vi "Connect.vi"(8 "error in (no error)":errorcluster, 11 "Stepper3D in":refnum<class "Stepper3D.lvclass">) -> (0 "error out":errorcluster, 3 "Stepper3D out":refnum<class "Stepper3D.lvclass">)   [LabVIEW 2014, in "Stepper3D.lvclass"]
uses:
  Stepper3D.lvclass
  Stepper3D.lvclass/Stepper3D.ctl
  Libs/stepper3D.lib/stepper3D.lvlib
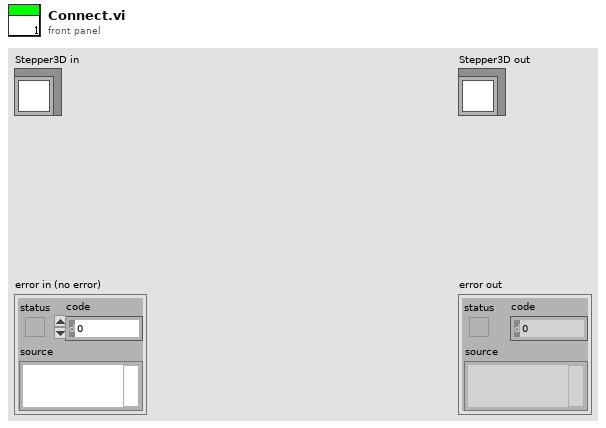
[diagram p1: front panel]
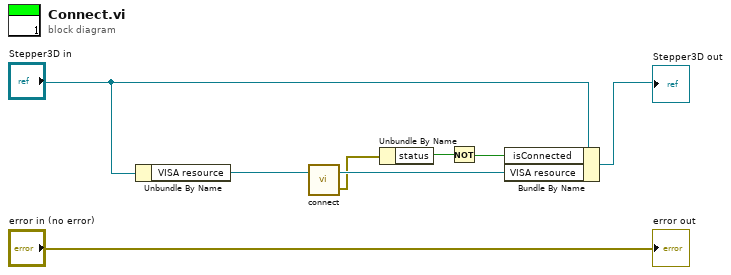
[diagram p0: block diagram]
diagram:
  n1 = Unbundle By Name("Stepper3D in") -> ("VISA resource"=w5:refnum<visa-resource-name>)
  n2 = call "connect.vi"("VISA resource name"=w5) -> ("error out"=w3:errorcluster, "VISA resource name out"=w4:refnum<visa-resource-name>)  [unwired: 1 in]
  n3 = Unbundle By Name(w3) -> ("status"=w1:bool)
  n4 = Not(x=w1) -> (.not. x?=w2:bool)
  n5 = Bundle By Name(cluster="Stepper3D in", "isConnected"=w2, "VISA resource"=w4) -> (→"Stepper3D out":refnum<class "Stepper3D.lvclass">)
  "error out" <- "error in (no error)"
